vi "DSA_Sync_Metrics.vi"() -> ()   [LabVIEW 2019]
uses:
  src/Instrument.DAQ/Typedefs/DAQ.Sampling.Sampling--Cluster.ctl
  src/Instrument.Lockin/Instrument.Lockin.lvclass
  src/Instrument.Lockin/Typedefs/Results Type--Enum.ctl
  src/Instrument.DAQ/Instrument.DAQ.lvclass
panel:
  out "Frequency (Hz)":dbl=13.0
  out "appended array":dbl[][](array[numeric])
  out "N":i32=97280
  out "XY Graph 3":cluster{dbl[], dbl[]}[](graph)
  in  "stop":bool
  out "Fs (Hz)":dbl=100.0
  out "XY Graph":cluster{i32[], dbl[]}[](graph)
  in  "Fs step":dbl=10000.0
  in  "Fs end":dbl=123456.0
  in  "Fs start":dbl=12345.0
  # "Sampling  frequency:"
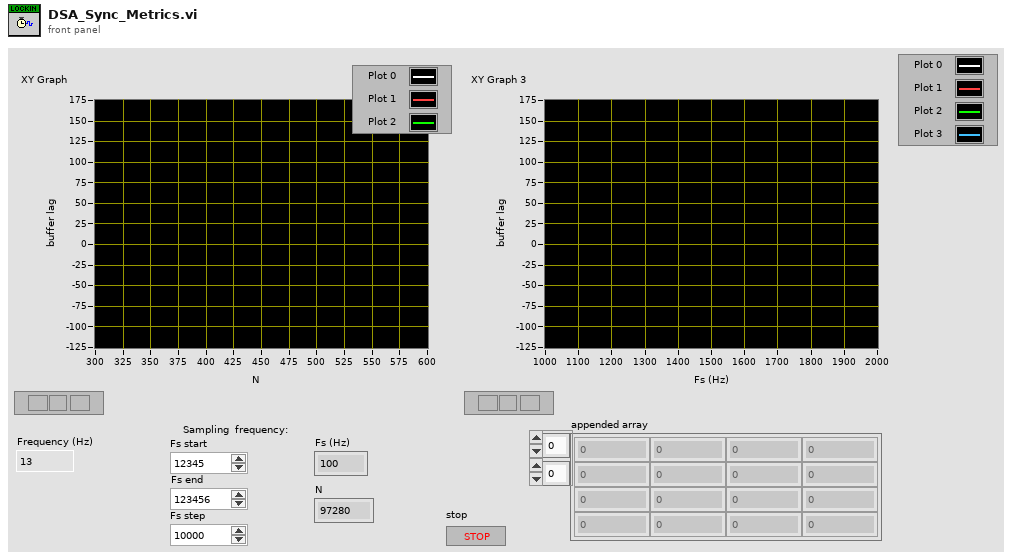
[diagram p1: front panel]
types:
  T1 = typedef "Instrument.Lockin.lvlib/Instrument.Lockin.lvclass/Results Type--Enum.ctl" = enum16{"X", "Y", "R", "Theta", "Mean"}
  T2 = typedef "Instrument.Lockin.lvlib/Instrument.DAQ.lvclass/DAQ.Sampling.Sampling--Cluster.ctl" = cluster{"Fs":dbl, "#s":i32}
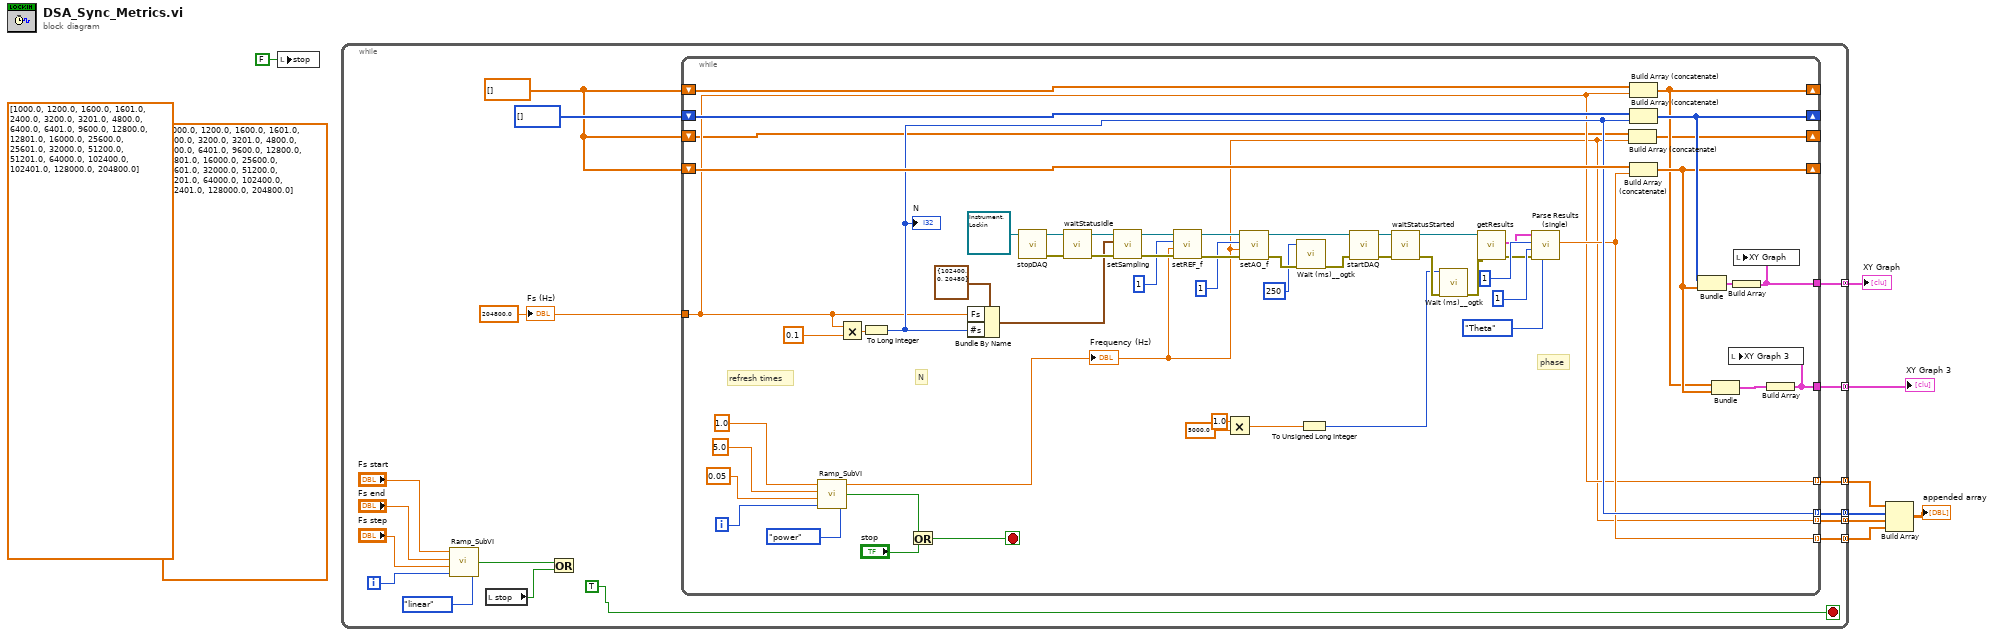
[diagram p0: block diagram]
diagram:
  (unwired) dbl[] [1000.0, 1200.0, 1600.0, 1601.0, 2400.0, 3200.0, 3201.0, 4800.0, 6400.0, 6401.0, 9600.0, 12800.0, 12801.0, 16000.0, 25600.0, 25601.0, 32000.0, 51200.0, 51201.0, 64000.0, 102400.0, 102401.0, 128000.0, 204800.0]
  (unwired) dbl[] [1000.0, 1200.0, 1600.0, 1601.0, 2400.0, 3200.0, 3201.0, 4800.0, 6400.0, 6401.0, 9600.0, 12800.0, 12801.0, 16000.0, 25600.0, 25601.0, 32000.0, 51200.0, 51201.0, 64000.0, 102400.0, 102401.0, 128000.0, 204800.0]
  n1 = local write "stop"(FALSE ("stop")) -> ()
  n2 = while {
    tunnel: [w22] -> w7 mode=concatenating
    tunnel: [w18] -> w6 mode=concatenating
    tunnel: [w16] -> w3 mode=concatenating
    tunnel: [w15] -> w4 mode=concatenating
    tunnel: [w14] -> w5 mode=concatenating
    tunnel: [w12] -> w1 mode=concatenating
    i -> [w24]
    stop <- TRUE stop-if-true
    w10 = 204800.0 ("Fs (Hz)")
    w13 = dbl[] []
    n3 = call <userlib>:"Ramp_SubVI.vi"("Enum"=enum16{"linear", "power"}."linear", "index"=w24, "step"="Fs step", "end"="Fs end", "start"="Fs start") -> ("Stop?"=w23:bool)  [unwired: 1 out]
    n4 = local read "stop"() -> (w11:bool)
    n5 = Or(x=w23, y=w11) -> ()  [unwired: 1 out]
    n6 = while {
      shift-right: [w73] -> _
      shift-left: w13 -> [w79]
      shift-right: [w70] -> _
      shift-left: w13 -> [w77]
      shift-right: [w74] -> _
      shift-left: i32[] [] -> [w78]
      tunnel: [w75] -> w22
      tunnel: w10 -> [w49]
      tunnel: [w71] -> w18
      tunnel: [w50] -> w16 mode=indexing
      tunnel: [w62] -> w15 mode=indexing
      tunnel: [w49] -> w14 mode=indexing
      shift-right: [w36] -> _
      shift-left: w13 -> [w35]
      tunnel: [w28] -> w12 mode=indexing
      i -> [w82]
      stop <- w27 stop-if-true
      # "N"
      # "phase"
      # "refresh times"
      n7 = call <userlib>:"Ramp_SubVI.vi"("Enum"=enum16{"linear", "power"}."power", "index"=w82, "step"=0.05 ("x"), "end"=5.0 ("x"), "start"=1.0 ("x")) -> ("Stop?"=w80:bool, "Numeric"=w28:dbl)
      "Frequency (Hz)" <- w28
      n8 = Multiply(x=w49, y=0.1 ("x")) -> (x*y=w59:dbl)
      n9 = To Long Integer(number=w59) -> (32bit integer=w62:i32)
      "N" <- w62
      n10 = Or(x=w80, y="stop") -> (x .or. y?=w27:bool)
      n11 = Bundle By Name(cluster=T2 {"Fs"=102400.0, "#s"=20480} ("Sampling"), "Fs"=w49, "#s"=w62) -> (w26:T2)
      n12 = call-dynamic "stopDAQ.vi"("Instrument.Lockin in"=refnum<class "Instrument.Lockin.lvclass"> refnum) -> ("error out"=w64:errorcluster, "Instrument.Lockin out"=w65:refnum<class "Instrument.Lockin.lvclass">)  [unwired: 9 in]
      n13 = call-dynamic "waitStatusIdle.vi"("error in (no error)"=w64, "Instrument.Lockin in"=w65) -> ("error out"=w61:errorcluster, "Instrument.Lockin out"=w60:refnum<class "Instrument.Lockin.lvclass">)  [unwired: 8 in]
      n14 = call-dynamic "setSampling.vi"("error in (no error)"=w61, "sampling"=w26, "Instrument.Lockin in"=w60) -> ("error out"=w41:errorcluster, "Instrument.Lockin out"=w40:refnum<class "Instrument.Lockin.lvclass">)  [unwired: 7 in]
      n15 = call-dynamic "setREF_f.vi"("error in (no error)"=w41, "Frequency (Hz)"=w28, "REF Channel"=1, "Instrument.Lockin in"=w40) -> ("error out"=w43:errorcluster, "Instrument.Lockin out"=w44:refnum<class "Instrument.Lockin.lvclass">)  [unwired: 6 in]
      n16 = Multiply(x=1.0, y=5000.0) -> (x*y=w58:dbl)
      n17 = call-dynamic "setAO_f.vi"("error in (no error)"=w43, "Frequency (Hz)"=w28, "AO Channel"=1, "Instrument.Lockin in"=w44) -> ("error out"=w34:errorcluster, "Instrument.Lockin out"=w46:refnum<class "Instrument.Lockin.lvclass">)  [unwired: 6 in]
      n18 = call <userlib>:"Wait (ms)__ogtk.vi"("error in (no error)"=w34, "milliseconds to wait"=u32 250) -> ("error out"=w32:errorcluster)  [unwired: 8 in, 1 out]
      n19 = To Unsigned Long Integer(number=w58) -> (unsigned 32bit integer=w31:u32)
      n20 = call-dynamic "startDAQ.vi"("error in (no error)"=w32, "Instrument.Lockin in"=w46) -> ("error out"=w38:errorcluster, "Instrument.Lockin out"=w47:refnum<class "Instrument.Lockin.lvclass">)  [unwired: 8 in]
      n21 = call-dynamic "waitStatusStarted.vi"("error in (no error)"=w38, "Instrument.Lockin in"=w47) -> ("error out"=w37:errorcluster, "Instrument.Lockin out"=w45:refnum<class "Instrument.Lockin.lvclass">)  [unwired: 8 in]
      n22 = call <userlib>:"Wait (ms)__ogtk.vi"("error in (no error)"=w37, "milliseconds to wait"=w31) -> ("error out"=w53:errorcluster)  [unwired: 8 in, 1 out]
      n23 = call-dynamic "getResults.vi"("error in (no error)"=w53, "Instrument.Lockin in"=w45) -> ("error out"=w52:errorcluster, "Results (Dictionary)"=w51:cluster{"key":string, "value":dbl}[])  [unwired: 6 in, 2 out]
      n24 = call "Parse Results (single).vi"("Datatype"=Results_Type--Enum."Theta" ("Type"), "error in (no error)"=w52, "Reference Channel"=1, "AI Channel"=1, "Results (Dictionary)"=w51) -> ("Data"=w50:dbl)  [unwired: 3 in, 3 out]
      n25 = Build Array (concatenate)(w35, w28) -> (w36:dbl[])
      n26 = Build Array (concatenate)(w77, w49) -> (w70:dbl[])
      n27 = Build Array (concatenate)(w78, w62) -> (w74:i32[])
      n28 = Build Array (concatenate)(w79, w50) -> (w73:dbl[])
      n29 = Bundle(w74, w73) -> (w76:cluster{i32[], dbl[]})  [unwired: 1 in]
      n30 = Bundle(w70, w73) -> (w72:cluster{dbl[], dbl[]})  [unwired: 1 in]
      n31 = Build Array(w76) -> (w75:cluster{i32[], dbl[]}[])
      n32 = local write "XY Graph"(w75) -> ()
      n33 = Build Array(w72) -> (w71:cluster{dbl[], dbl[]}[])
      n34 = local write "XY Graph 3"(w71) -> ()
    }
    "Fs (Hz)" <- w10
  }
  "XY Graph" <- w7
  "XY Graph 3" <- w6
  n35 = Build Array(w5, w4, w1, w3) -> (→"appended array":dbl[][])
